vi "Update WebView2 Assembly.vi"   [LabVIEW 2020]
uses:
  WebView2 Updater/WebView2 Updater.lvclass
types:
  T1 = enum32{"Invalid", "Standard", "Closed", "Hidden", "Minimized", "Maximized"}
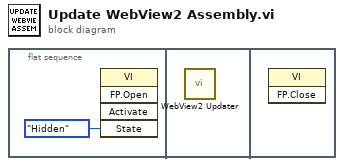
[diagram p0: block diagram]
diagram:
  n1 = flat-sequence {
    frame #0 {
      n2 = invoke class="VI" method="FP.Open"("State"=T1."Hidden") -> ()  [unwired: 4 in, 5 out]
    }
    frame #1 {
      n3 = call "WebView2 Updater.vi"() -> ()  [unwired: 12 in]
    }
    frame #2 {
      n4 = invoke class="VI" method="FP.Close"() -> ()  [unwired: 3 in, 3 out]
    }
  }
